vi "Barcode Reprint.vi"() -> ()   [LabVIEW 2020]
uses:
  <vilib>/Utility/miscctls.llb/LVRowAndColumnUnsignedTypeDef.ctl
panel:
  in  "Reprint":bool
  out "element 4":string
  out "element 3":string
  out "element 2":string
  out "element":string
  in  "Final Table":i32(listbox)
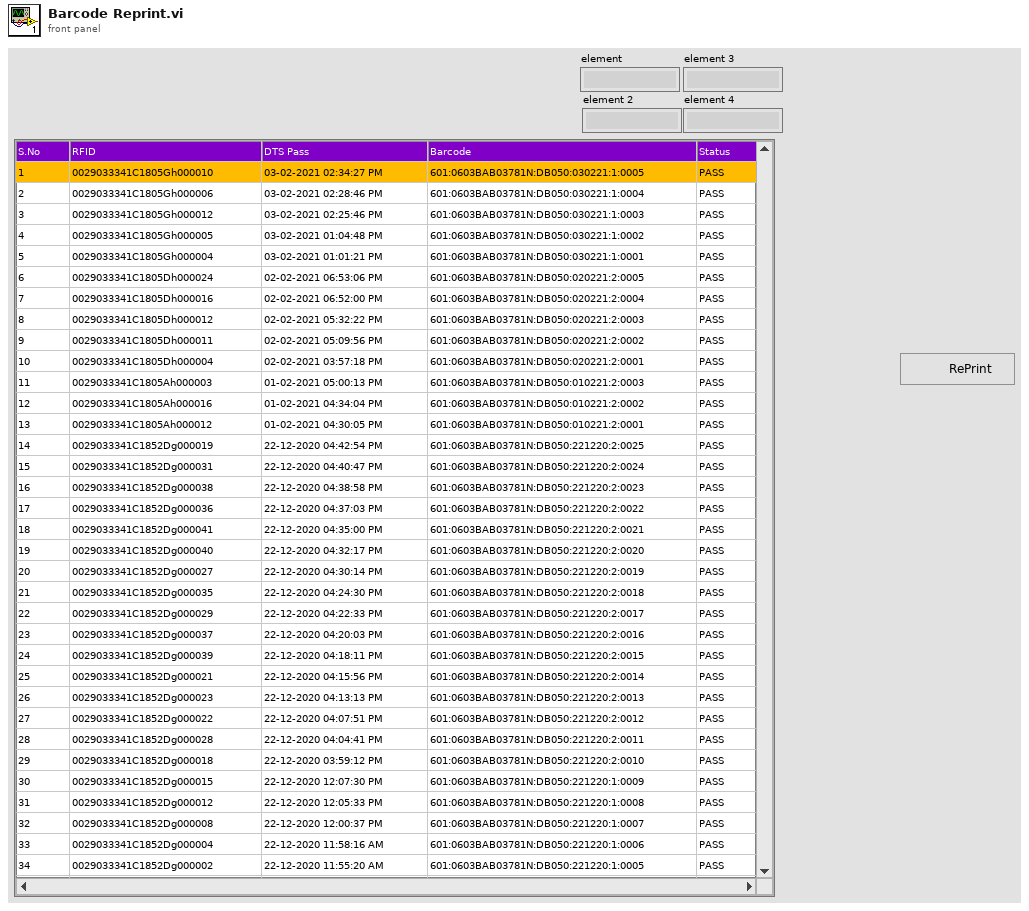
[diagram p1: front panel]
types:
  T1 = typedef "LVRowAndColumnUnsignedTypeDef.ctl" = cluster{"Row":u32, "Column":u32}
  T2 = typedef "TD SQL.ctl" = cluster{"MS SQL Connection":T3, "UDL File":path, "Remarks Ref.":refnum<vi>, "Time":string, "DCODE":string, "WIP+1":i64, "MC No?":i32, "POKAYOKE?":bool, "Expected Result":string, "Result [Status]":string, "Clock":dbl, "RFID":string, "WIP Queue":refnum<queue>}
  T3 = typedef "NI_Database_API.lvlib/Conn ObjectReference.ctl" = refnum<k1>
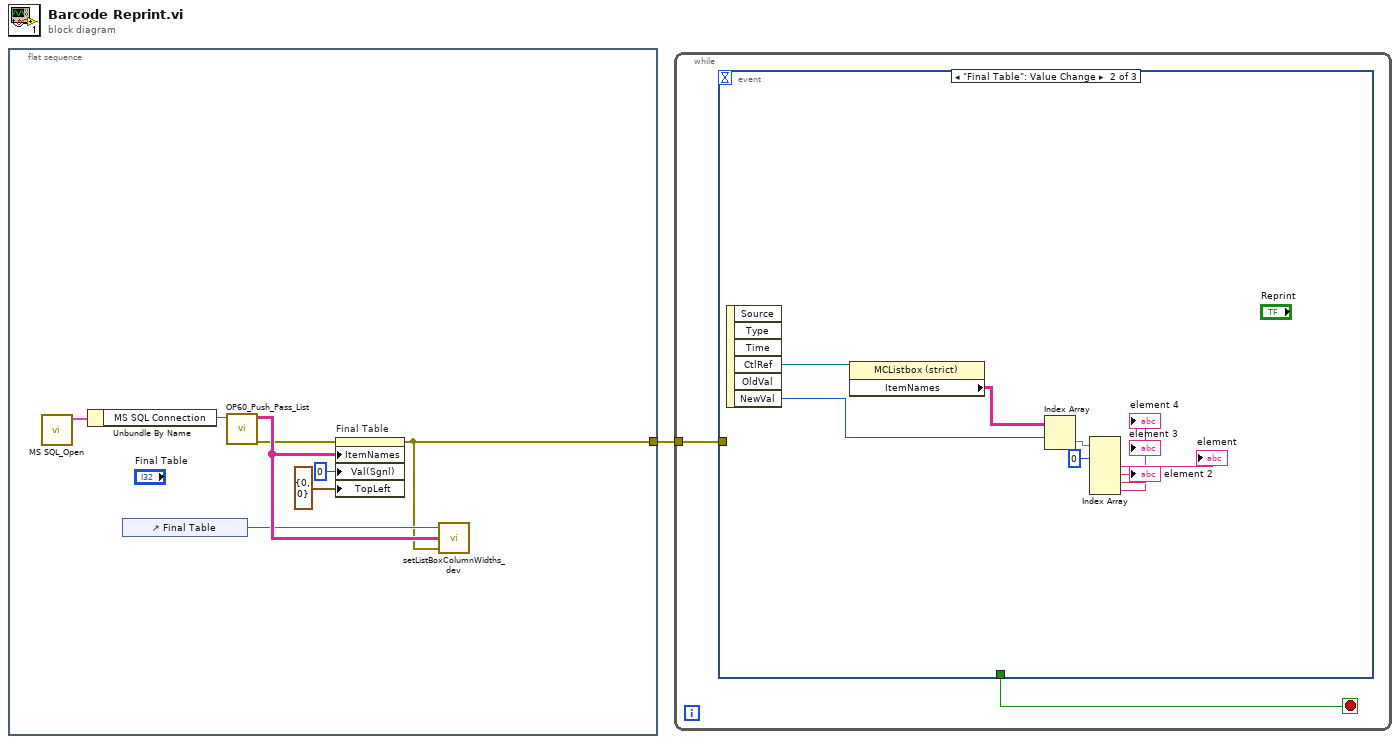
[diagram p0: block diagram]
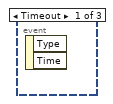
[diagram p2: hidden frame]
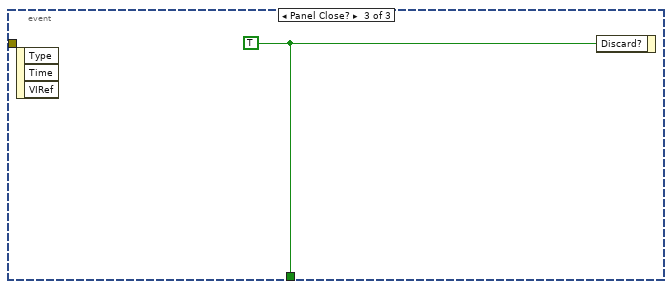
[diagram p3: hidden frame]
diagram:
  n1 = flat-sequence {
    tunnel: [w2] -> w1
    frame #0 {
      n2 = call "MS SQL_Open.vi"() -> ("Ref Out"=w9:T2)  [unwired: 9 in, 2 out]
      n3 = Unbundle By Name(w9) -> ("MS SQL Connection"=w8:T3)
      n4 = control-ref of="Final Table"() -> (w6:refnum<vi>)
      n5 = call "OP60_Push_Pass_List.vi"("Refnum in"=w8) -> ("error out"=w5:errorcluster, "Array"=w7:string[][])  [unwired: 9 in]
      n6 = property on="Final Table" class="MCListbox (strict)"(error in=w5, "ItemNames"=w7, "Val(Sgnl)"=0 ("Final Table"), "TopLeft"=T1 {"Row"=0, "Column"=0} ("Top Left Visible Cell")) -> (error out=w2:errorcluster)  [unwired: 1 in, 1 out]
      n7 = call "setListBoxColumnWidths_dev.vi"("error in (no error)"=w2, "table data"=w7, "MCListbox Refnum"=w6) -> ()
    }
  }
  n8 = while {
    tunnel: w1 -> [w10]
    stop <- w11 stop-if-true
    n9 = event shown="[1] \"Final Table\": Value Change" {
      selector: _ -> [_ _ _]
      dyn-events: _ -> [_ _ _]
      timeout: _ -> [_ _ _]
      tunnel: [_ _ w21] -> w11
      tunnel: w10 -> [_ _ _]
      event Timeout {
        n10 = event-data() -> ()  [unwired: 1 in, 2 out]
      }
      event "Final Table": Value Change {
        n11 = event-data() -> ("CtlRef"=w20:refnum<vi>, "NewVal"=w18:i32)  [unwired: 1 in, 4 out]
        n12 = property class="MCListbox (strict)"(reference=w20) -> ("ItemNames"=w19:string[][])  [unwired: 1 in, 2 out]
        n13 = Index Array(array=w19, index (row)=w18) -> (element=w17:string[])  [unwired: 1 in]
        n14 = Index Array(array=w17, index #1=0 ("index")) -> (element #2=→"element":string, element #3=→"element 2":string, element #4=→"element 3":string, element #5=→"element 4":string)  [unwired: 4 in, 1 out]
      }
      event Panel Close? {
        w21 = TRUE ("Discard?")
        n15 = event-data() -> ()  [unwired: 1 in, 3 out]
        n16 = event-data("Discard?"=w21) -> ()  [unwired: 1 in, 1 out]
      }
    }
  }
